vi "Descanner1_counter.vi"(0 "Pix":i32, 1 "scanPix":i32, 2 "delta_p":i32, 3 "Data":i64[](array[numeric]), 4 "last_count prev line":i64) -> (5 "2Lines":i64[][](array[numeric]), 6 "last_count":i64)   [LabVIEW 2016]
panel:
  out "Waveform Graph":i64[](graph)
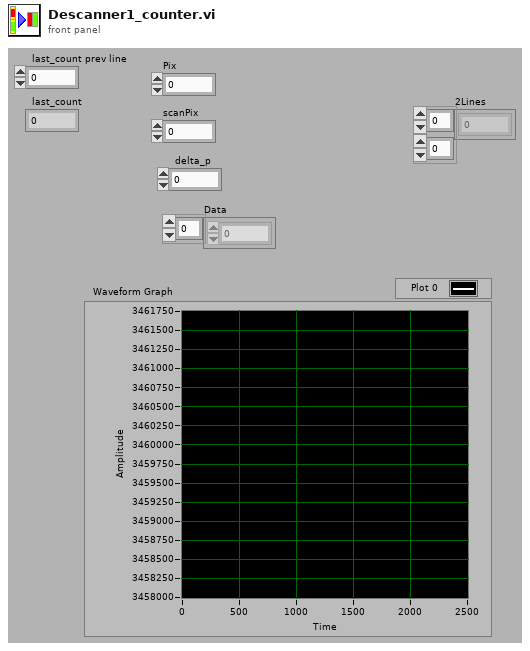
[diagram p1: front panel]
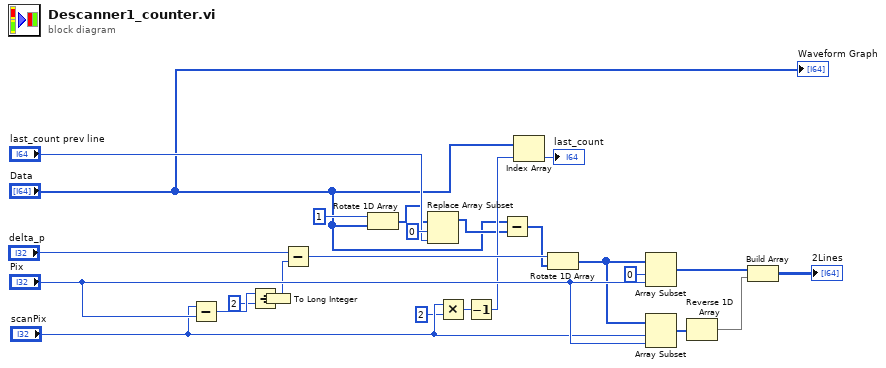
[diagram p0: block diagram]
diagram:
  n1 = Subtract(x="scanPix", y="Pix") -> (x-y=w25:i32)
  n2 = Divide(x=w25, y=2) -> (x/y=w8:dbl)
  n3 = To Long Integer(number=w8) -> (32bit integer=w3:i32)
  n4 = Subtract(x="delta_p", y=w3) -> (x-y=w20:i32)
  n5 = Rotate 1D Array(1:"Data", 2:1 ("n")) -> (0:w6:i64[])
  n6 = Replace Array Subset(array=w6, new element="last_count prev line", index=0) -> (w5:i64[])
  n7 = Multiply(x="scanPix", y=2) -> (x*y=w11:i32)
  n8 = Decrement(x=w11) -> (x-1=w10:i32)
  n9 = Subtract(x="Data", y=w5) -> (x-y=w4:i64[])
  n10 = Index Array(array="Data", index=w10) -> (element=→"last_count":i64)
  n11 = Rotate 1D Array(1:w4, 2:w20) -> (0:w7:i64[])
  n12 = Array Subset(array=w7, index=0, length="Pix") -> (w9:i64[])
  n13 = Array Subset(array=w7, index="scanPix", length="Pix") -> (w21:i64[])
  n14 = Reverse 1D Array(array=w21) -> (reversed array=w18:i64[])
  n15 = Build Array(w9, w18) -> (→"2Lines":i64[][])
  "Waveform Graph" <- "Data"
